vi "Main.vi"() -> ()   [LabVIEW 2018, in "Timer Module.lvlib"]
doc: "This template is based off of the Queued Message Handler design pattern and the Queued Message Handler project template that ships with LabVIEW.\n\nThe main difference is that the queue is private to this module and communication between modules is performed via Broadcast and Request events.\n\nRequest events are wrapped in public API methods and are handled in the Event Handling Loop (EHL) of this VI. Any module can register for Broadcast events sent by this module. The EHL generates messages based on user interface actions.\n\nThe Message Handling Loop (MHL) processes messages generated by the EHL, or by other messages. The messages are string values, so new messages can be added easily to the Message Cases case structure in the MHL. Each message cluster can also provide an optional value for Message Data, which is a variant that can be converted to whatever message-specific data is required.\n_____\nBased on Delacor QMH Project Template 4.1.0.56."
uses:
  Timer Module.lvlib
  <vilib>/Delacor/Delacor QMH/Libraries/Cloneable Module Admin_class/Delacor_lib_QMH_Cloneable Module Admin.lvclass
  C:/Program Files (x86)/National Instruments/LabVIEW 2018/vi.lib/Delacor/Delacor QMH/Libraries/Module Admin_class/Delacor_lib_QMH_Module Admin.lvclass
  Module Data--cluster.ctl
  <vilib>/Delacor/Delacor QMH/Libraries/Cloneable Module Admin_class/Delacor_lib_QMH_Cloneable Module Admin.lvclass/Delacor_lib_QMH_Cloneable Module Admin.ctl
  Stop Argument--cluster.ctl
  <vilib>/Delacor/Delacor QMH/Libraries/Module Admin_class/Delacor_lib_QMH_Module Admin.lvclass/Delacor_lib_QMH_Module Admin.ctl
  Start Timer Argument--cluster.ctl
  <vilib>/Utility/miscctls.llb/LVPointTypeDef.ctl
  <vilib>/Delacor/Delacor QMH/Libraries/Cloneable Module Admin_class/Delacor_lib_QMH_Get Module ID.vi
  <vilib>/Delacor/Delacor QMH/Libraries/Module Admin_class/Delacor_lib_QMH_Get External Launch.vi
  <vilib>/Delacor/Delacor QMH/Libraries/Message Queue_class/Delacor_lib_QMH_Enqueue Message (Single).vi
  <vilib>/Utility/error.llb/Error Cluster From Error Code.vi
  <vilib>/ErrorRing/Error Ring.xnode
  <vilib>/Delacor/Delacor QMH/Libraries/Message Queue_class/Delacor_lib_QMH_Message Queue.lvclass
  Clone Registration/Clone Registration.lvlib
panel:
  out "Timer":timestamp format="%^<%H:%M:%S%3u>T"
  out "error out":errorcluster
  in  "Module Admin":refnum<class "Delacor_lib_QMH_Cloneable Module Admin.lvclass">
  out "Status":string
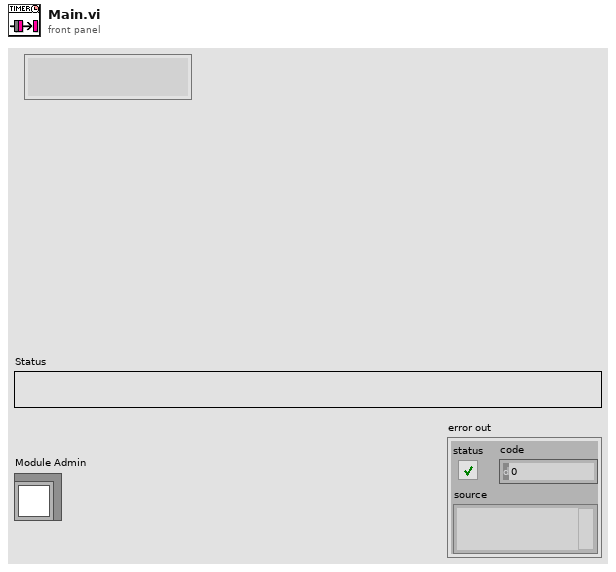
[diagram p1: front panel]
types:
  T1 = typedef "Timer Module.lvlib/Request Events--cluster.ctl" = cluster{"Stop Module":refnum<user-event>, "Show Panel":refnum<user-event>, "Hide Panel":refnum<user-event>, "Show Diagram":refnum<user-event>, "Get Module Execution Status":refnum<user-event>, "Start Timer":refnum<user-event>, "Pause Timer":refnum<user-event>, "Unpause Timer":refnum<user-event>}
  T2 = typedef "Timer Module.lvlib/Module Data--cluster.ctl" = cluster{"Status":string}
  T3 = enum32{"invalid lock state", "Not Locked", "Locked (No Password)", "Password-protected"}
  T4 = typedef "Timer Module.lvlib/Stop Argument--cluster.ctl" = cluster{"Module ID":i32, "Origin":string, "Exit via Stop Module Req?":bool, "Wait for Module to stop?":bool}
  T5 = typedef "Timer Module.lvlib/Start Timer Argument--cluster.ctl" = cluster{"Module ID":i32, "Boolean":bool}
  T6 = typedef "LVPointTypeDef.ctl" = cluster{"Horizontal":i16, "Vertical":i16}
  T7 = enum32{"Invalid", "Standard", "Closed", "Hidden", "Minimized", "Maximized"}
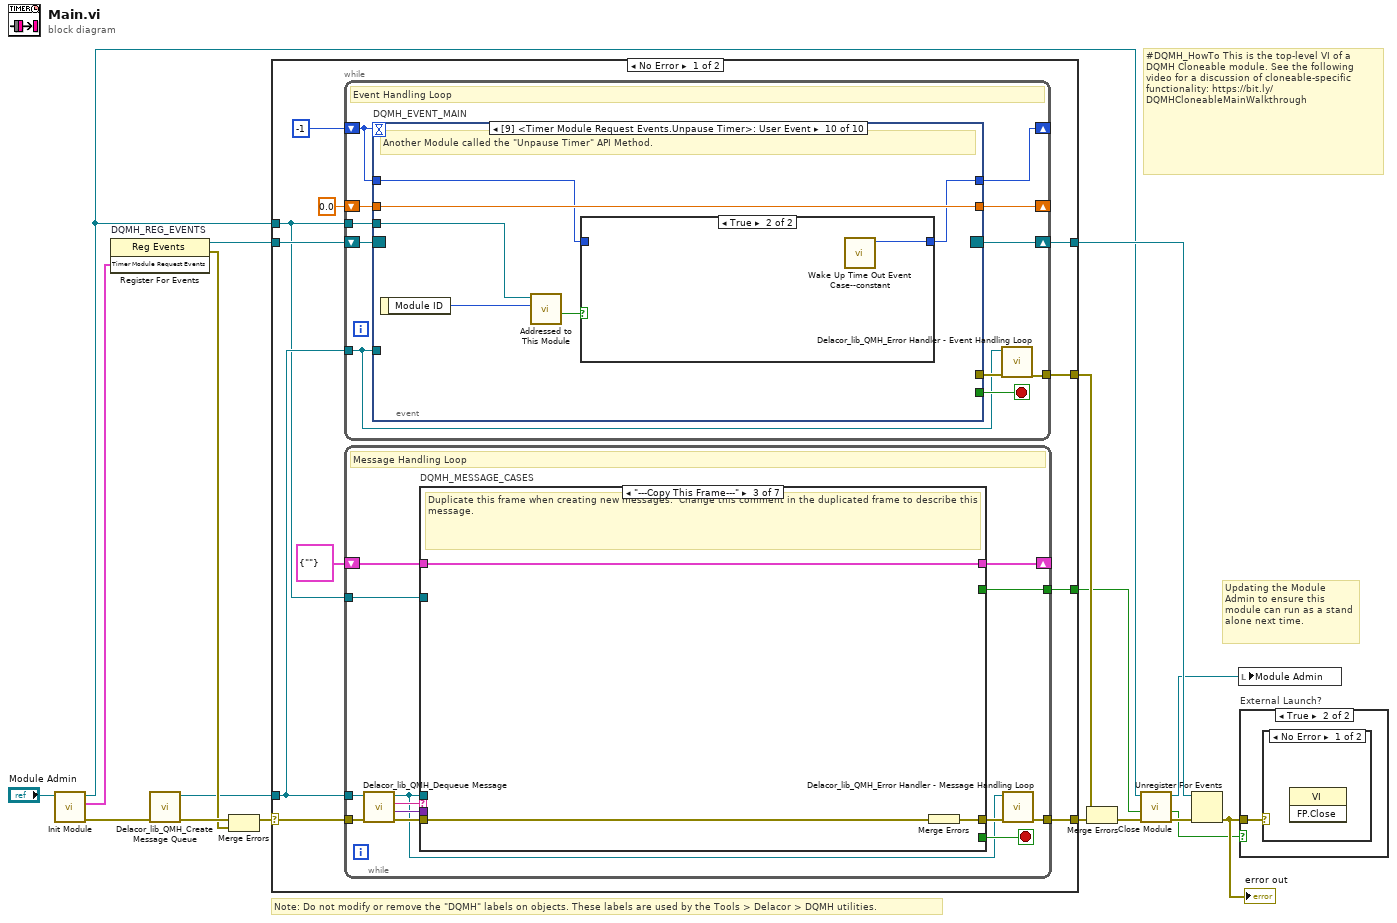
[diagram p0: block diagram]
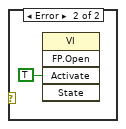
[diagram p3: hidden frame]
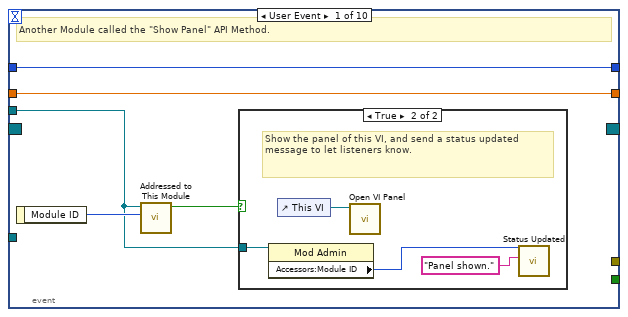
[diagram p4: hidden frame]
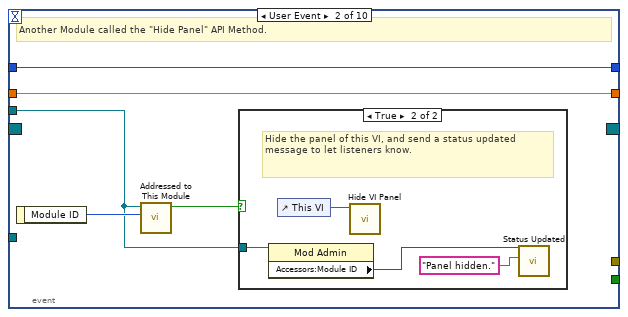
[diagram p6: hidden frame]
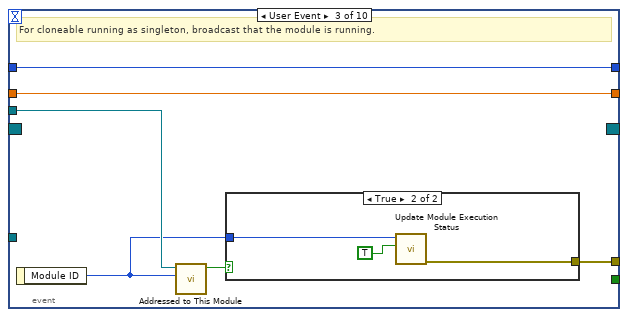
[diagram p8: hidden frame]
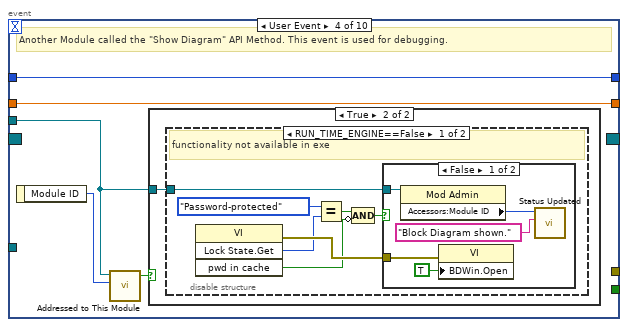
[diagram p10: hidden frame]
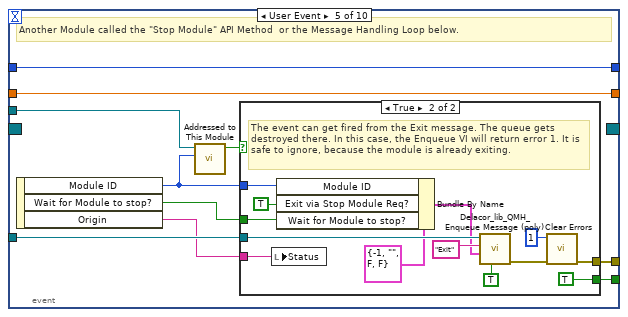
[diagram p14: hidden frame]
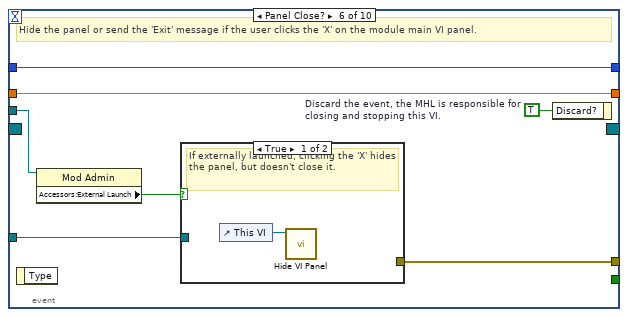
[diagram p16: hidden frame]
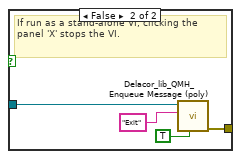
[diagram p17: hidden frame]
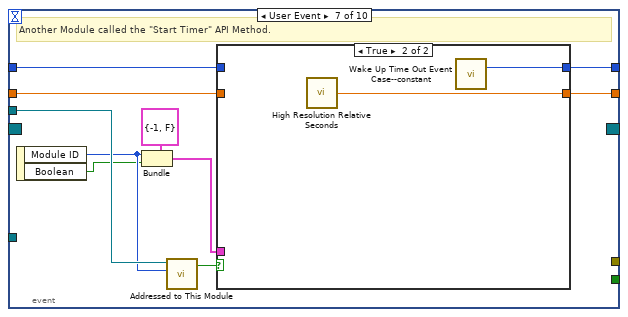
[diagram p18: hidden frame]
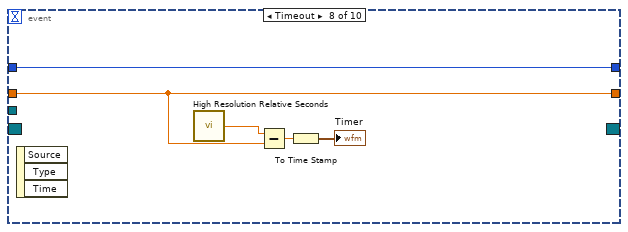
[diagram p20: hidden frame]
diagram:
  # "#DQMH_HowTo This is the top-level VI of a DQMH Cloneable module. See the following video for a discussion of cloneable-specific functionality: https://bit.ly/DQMHCloneableMainWalkthrough"
  # "Note: Do not modify or remove the \"DQMH\" labels on objects. These labels are used by the Tools > Delacor > DQMH utilities."
  # "Updating the Module Admin to ensure this module can run as a stand alone next time."
  n1 = call "Init Module.vi"("Cloneable Module Admin in"="Module Admin") -> ("error out"=w15:errorcluster, "Timer Module Request Events"=w7:T1, "Cloneable Module Admin out"=w4:refnum<class "Delacor_lib_QMH_Cloneable Module Admin.lvclass">)  [unwired: 8 in]
  n2 = register-events "DQMH_REG_EVENTS"(w7) -> (reference out=w8:refnum<event-registration>, error out=w10:errorcluster)  [unwired: 2 in]
  n3 = call <vilib>:"Delacor_lib_QMH_Create Message Queue.vi"("error in (no error)"=w15) -> ("error out"=w12:errorcluster, "Message Queue"=w6:refnum<class "Delacor_lib_QMH_Message Queue.lvclass">)  [unwired: 9 in]
  n4 = Merge Errors(w12, w10) -> (w11:errorcluster)
  n5 = case shown="No Error" w11 {
    selector: w11 -> [w27 w253]
    tunnel: [w29 w253] -> w16
    tunnel: [w26 w252] -> w9
    tunnel: w8 -> [w24 w252]
    tunnel: w6 -> [w23 _]
    tunnel: [w28 _] -> w17
    tunnel: w4 -> [w22 w248]
    tunnel: [w21 _] -> w2
    frame No Error {
      n6 = while {
        tunnel: w23 -> [w34]
        shift-right: [w37] -> w26
        shift-left: w24 -> [w38]
        tunnel: [w39] -> w28
        tunnel: w22 -> [w35]
        shift-right: [w33] -> _
        shift-left: -1 -> [w32]
        shift-right: [w31] -> _
        shift-left: 0.0 ("relative seconds") -> [w30]
        stop <- w36 stop-if-true
        # "Event Handling Loop"
        n7 = event "DQMH_EVENT_MAIN" shown="[9] <Timer Module Request Events.Unpause Timer>: User Event" {
          selector: w38 -> [_ _ _ _ _ _ _ _ _ _]
          dyn-events: [_ _ _ _ _ _ _ _ _ _] -> w37
          timeout: w32 -> [_ _ _ _ _ _ _ _ _ _]
          tunnel: [_ _ _ _ w91 _ _ _ _ _] -> w36
          tunnel: w34 -> [_ _ _ _ w94 w112 _ _ _ _]
          tunnel: [_ _ w64 _ w95 w115 _ _ _ _] -> w40
          tunnel: w35 -> [w43 w52 w62 w70 w93 w113 w129 _ w143 w151]
          tunnel: [w42 w51 w60 w69 w87 w110 w123 w139 w140 w148] -> w33
          tunnel: w32 -> [w42 w51 w60 w69 w87 w110 w124 w139 w141 w149]
          tunnel: [w41 w50 w59 w68 w86 w109 w122 w137 w145 w153] -> w31
          tunnel: w30 -> [w41 w50 w59 w68 w86 w109 w121 w137 w145 w153]
          event User Event {
            # "Another Module called the \"Show Panel\" API Method."
            n8 = event-data() -> ("Module ID"=w44:i32)  [unwired: 1 in]
            n9 = call "Addressed to This Module.vi"("Module ID from Argument"=w44, "Module Admin"=w43) -> ("Addressed to this instance?"=w45:bool)  [unwired: 8 in, 1 out]
            n10 = case shown="True" w45 {
              tunnel: w43 -> [_ w47]
              frame False {
              }
              frame True {
                # "Show the panel of this VI, and send a status updated message to let listeners know."
                n11 = property class="Mod Admin"(reference=w47) -> ("Accessors:Module ID"=w46:i32)  [unwired: 1 in, 2 out]
                n12 = control-ref of="This VI"() -> (w49:refnum<vi>)
                n13 = call "Open VI Panel.vi"("VI"=w49) -> ()  [unwired: 10 in, 1 out]
                n14 = call "Status Updated.vi"("Status"="Panel shown." ("format string"), "Module ID"=w46) -> ()  [unwired: 9 in, 1 out]
              }
            }
          }
          event User Event {
            # "Another Module called the \"Hide Panel\" API Method."
            n15 = event-data() -> ("Module ID"=w53:i32)  [unwired: 1 in]
            n16 = call "Addressed to This Module.vi"("Module ID from Argument"=w53, "Module Admin"=w52) -> ("Addressed to this instance?"=w54:bool)  [unwired: 8 in, 1 out]
            n17 = case shown="True" w54 {
              tunnel: w52 -> [_ w56]
              frame False {
              }
              frame True {
                # "Hide the panel of this VI, and send a status updated message to let listeners know."
                n18 = property class="Mod Admin"(reference=w56) -> ("Accessors:Module ID"=w55:i32)  [unwired: 1 in, 2 out]
                n19 = control-ref of="This VI"() -> (w58:refnum<vi>)
                n20 = call "Hide VI Panel.vi"("VI"=w58) -> ()  [unwired: 10 in, 1 out]
                n21 = call "Status Updated.vi"("Status"="Panel hidden." ("format string"), "Module ID"=w55) -> ()  [unwired: 9 in, 1 out]
              }
            }
          }
          event User Event {
            # "For cloneable running as singleton, broadcast that the module is running."
            n22 = event-data() -> ("Module ID"=w61:i32)  [unwired: 1 in]
            n23 = call "Addressed to This Module.vi"("Module ID from Argument"=w61, "Module Admin"=w62) -> ("Addressed to this instance?"=w63:bool)  [unwired: 8 in, 1 out]
            n24 = case shown="True" w63 {
              tunnel: [_ w67] -> w64
              tunnel: w61 -> [_ w66]
              frame False {
              }
              frame True {
                n25 = call "Update Module Execution Status.vi"("Running?"=TRUE, "Module ID"=w66) -> ("error out"=w67:errorcluster)  [unwired: 9 in]
              }
            }
          }
          event User Event {
            # "Another Module called the \"Show Diagram\" API Method. This event is used for debugging."
            n26 = event-data() -> ("Module ID"=w71:i32)  [unwired: 1 in]
            n27 = call "Addressed to This Module.vi"("Module ID from Argument"=w71, "Module Admin"=w70) -> ("Addressed to this instance?"=w72:bool)  [unwired: 8 in, 1 out]
            n28 = case shown="True" w72 {
              tunnel: w70 -> [_ w73]
              frame False {
              }
              frame True {
                n29 = disable-structure shown="RUN_TIME_ENGINE==False" {
                  disable-tunnel: w73 -> [w74 _]
                  frame condition #0 (active) {
                    # "functionality not available in exe"
                    n30 = invoke class="VI" method="Lock State.Get"() -> (error out=w80:errorcluster, "Get Lock State"=w79:T3, "pwd in cache"=w76:bool)  [unwired: 4 in, 1 out]
                    n31 = Equal?(x=T3."Password-protected", y=w79) -> (x = y?=w77:bool)
                    n32 = Compound Arithmetic op=AND(w77, invert w76) -> (w75:bool)
                    n33 = case shown="False" w75 {
                      tunnel: w80 -> [w85 _]
                      tunnel: w74 -> [w82 _]
                      frame False {
                        n34 = property class="Mod Admin"(reference=w82) -> ("Accessors:Module ID"=w81:i32)  [unwired: 1 in, 2 out]
                        n35 = property class="VI"(error in=w85, "BDWin.Open"=TRUE ("Block Diagram Window:Open")) -> ()  [unwired: 1 in, 2 out]
                        n36 = call "Status Updated.vi"("Status"="Block Diagram shown." ("format string"), "Module ID"=w81) -> ()  [unwired: 9 in, 1 out]
                      }
                      frame True {
                        # "Password-protected VI, and the password is not in the cache. Do not show the diagram."
                      }
                    }
                  }
                  frame condition #1 {
                  }
                }
              }
            }
          }
          event User Event {
            # "Another Module called the \"Stop Module\" API Method  or the Message Handling Loop below."
            n37 = event-data() -> ("Module ID"=w89:i32, "Wait for Module to stop?"=w90:bool, "Origin"=w88:string)  [unwired: 1 in]
            n38 = call "Addressed to This Module.vi"("Module ID from Argument"=w89, "Module Admin"=w93) -> ("Addressed to this instance?"=w92:bool)  [unwired: 8 in, 1 out]
            n39 = case shown="True" w92 {
              tunnel: [_ w107] -> w95
              tunnel: w94 -> [_ w103]
              tunnel: [_ TRUE] -> w91
              tunnel: w90 -> [_ w98]
              tunnel: w89 -> [_ w100]
              tunnel: w88 -> [_ w96]
              frame False {
              }
              frame True {
                # "The event can get fired from the Exit message. The queue gets destroyed there. In this case, the Enqueue VI will return error 1. It is safe to ignore, because the module is already exiting."
                n40 = local write "Status"(w96) -> ()
                n41 = Bundle By Name(cluster=T4 {"Module ID"=-1, "Origin"="", "Exit via Stop Module Req?"=FALSE, "Wait for Module to stop?"=FALSE} ("Stop Argument"), "Module ID"=w100, "Exit via Stop Module Req?"=TRUE, "Wait for Module to stop?"=w98) -> (w97:T4)
                n42 = call-poly <vilib>:"Delacor_lib_QMH_Enqueue Message (poly).vi"("Priority Message? (F)"=TRUE, "Message Data"=w97, "Message"="Exit", "Message Queue in"=w103) -> ("error out"=w108:errorcluster)  [unwired: 6 in, 1 out]
                n43 = call <vilib>:"Clear Errors.vi"("error in (no error)"=w108, "specific error code to clear (0: all)"=1) -> ("error out"=w107:errorcluster)  [unwired: 4 in, 1 out]
              }
            }
          }
          event Panel Close? {
            w114 = TRUE  # Discard the event, the MHL is responsible for closing and stopping this VI.
            # "Hide the panel or send the 'Exit' message if the user clicks the 'X' on the module main VI panel."
            n44 = event-data() -> ()  [unwired: 1 in, 1 out]
            n45 = property class="Mod Admin"(reference=w113) -> ("Accessors:External Launch"=w111:bool)  [unwired: 1 in, 2 out]
            n46 = case shown="True" w111 {
              tunnel: w112 -> [_ w119]
              tunnel: [_ w120] -> w115
              frame True {
                # "If externally launched, clicking the 'X' hides the panel, but doesn't close it."
                n47 = control-ref of="This VI"() -> (w116:refnum<vi>)
                n48 = call "Hide VI Panel.vi"("VI"=w116) -> ()  [unwired: 10 in, 1 out]
              }
              frame False {
                # "If run as a stand-alone VI, clicking the panel 'X' stops the VI."
                n49 = call-poly <vilib>:"Delacor_lib_QMH_Enqueue Message (poly).vi"("Priority Message? (F)"=TRUE, "Message"="Exit", "Message Queue in"=w119) -> ("error out"=w120:errorcluster)  [unwired: 7 in, 1 out]
              }
            }
            n50 = event-data("Discard?"=w114) -> ()  [unwired: 1 in, 1 out]
          }
          event User Event {
            # "Another Module called the \"Start Timer\" API Method."
            n51 = event-data() -> ("Module ID"=w126:i32, "Boolean"=w125:bool)  [unwired: 1 in]
            n52 = Bundle(cluster=T5 {"Module ID"=-1, "Boolean"=FALSE} ("Start Timer Argument"), "Module ID"=w126, "Boolean"=w125) -> (w127:T5)
            n53 = call "Addressed to This Module.vi"("Module ID from Argument"=w126, "Module Admin"=w129) -> ("Addressed to this instance?"=w130:bool)  [unwired: 8 in, 1 out]
            n54 = case shown="True" w130 {
              tunnel: w127 -> [_ _]
              tunnel: w124 -> [w132 _]
              tunnel: [w132 w134] -> w123
              tunnel: [w131 w133] -> w122
              tunnel: w121 -> [w131 _]
              frame False {
              }
              frame True {
                n55 = call <vilib>:"High Resolution Relative Seconds.vi"() -> ("relative seconds"=w133:dbl)
                n56 = call "Wake Up Time Out Event Case--constant.vi"() -> ("Wake up TimeOut Event Case"=w134:i32)  [unwired: 11 in]
              }
            }
          }
          event Timeout {
            n57 = event-data() -> ()  [unwired: 1 in, 3 out]
            n58 = call <vilib>:"High Resolution Relative Seconds.vi"() -> ("relative seconds"=w138:dbl)
            n59 = Subtract(x=w138, y=w137) -> (x-y=w136:dbl)
            n60 = To Time Stamp(1:w136) -> (0:→"Timer":timestamp)
          }
          event User Event {
            # "Another Module called the \"Pause Timer\" API Method."
            n61 = event-data() -> ("Module ID"=w142:i32)  [unwired: 1 in]
            n62 = call "Addressed to This Module.vi"("Module ID from Argument"=w142, "Module Admin"=w143) -> ("Addressed to this instance?"=w144:bool)  [unwired: 8 in, 1 out]
            n63 = case shown="True" w144 {
              tunnel: w141 -> [w146 _]
              tunnel: [w146 w147] -> w140
              frame False {
              }
              frame True {
                w147 = -1  # Put TimeOut event case to sleep
              }
            }
          }
          event User Event {
            # "Another Module called the \"Unpause Timer\" API Method."
            n64 = event-data() -> ("Module ID"=w150:i32)  [unwired: 1 in]
            n65 = call "Addressed to This Module.vi"("Module ID from Argument"=w150, "Module Admin"=w151) -> ("Addressed to this instance?"=w152:bool)  [unwired: 8 in, 1 out]
            n66 = case shown="True" w152 {
              tunnel: [w154 w155] -> w148
              tunnel: w149 -> [w154 _]
              frame False {
              }
              frame True {
                n67 = call "Wake Up Time Out Event Case--constant.vi"() -> ("Wake up TimeOut Event Case"=w155:i32)  [unwired: 11 in]
              }
            }
          }
        }
        n68 = call-dynamic "Delacor_lib_QMH_Error Handler - Event Handling Loop.vi"("error in (no error)"=w40, "Message Queue in"=w34) -> ("dup error in"=w39:errorcluster)  [unwired: 8 in, 1 out]
      }
      n69 = while {
        tunnel: w23 -> [w159]
        shift-right: [w163] -> _
        shift-left: T2 {"Status"=""} ("Data Cluster") -> [w164]
        tunnel: w27 -> [w167]
        tunnel: [w165] -> w29
        tunnel: w22 -> [w157]
        tunnel: [w156] -> w21
        stop <- w162 stop-if-true
        # "Message Handling Loop"
        n70 = call-dynamic "Delacor_lib_QMH_Dequeue Message.vi"("error in (no error)"=w167, "Message Queue in"=w159) -> ("error out"=w166:errorcluster, "Message Data"=w160:variant, "Message"=w161:string, "Message Queue out"=w158:refnum<class "Delacor_lib_QMH_Message Queue.lvclass">)  [unwired: 6 in]
        n71 = case "DQMH_MESSAGE_CASES" shown="\"---Copy This Frame---\"" w161 {
          selector: w161 -> [_ _ _ _ _ _ w233]
          tunnel: w158 -> [_ _ _ _ w197 w223 _]
          tunnel: w166 -> [w187 w191 w194 w196 w207 w229 w235]
          tunnel: [w185 w191 w193 w196 w203 w226 w236] -> w168
          tunnel: w164 -> [w178 w190 w192 w195 w202 w222 w234]
          tunnel: [w177 w190 w192 w195 w202 w222 w234] -> w163
          tunnel: [_ _ _ _ _ w221 _] -> w162
          tunnel: w160 -> [_ _ _ _ w201 w219 _]
          tunnel: w157 -> [w172 _ _ _ w200 w215 w231]
          tunnel: [_ _ _ _ _ w217 _] -> w156
          frame "Initialize" {
            w169 = "Initial Message" ("Initial Message")
            # "#CodeNeeded - Initialize the appearance of the front panel."
            # "#CodeNeeded - Initialize your state data here."
            # "Initialize - Any operation that needs to be done before the module can receive messages. Synchronize Caller Events.vi will inform Start Module.vi that the module has launched and is ready to receive messages. Module Did Init.vi will broadcast that the module initialized."
            n72 = call "Synchronize Caller Events.vi"("error in (no error)"=w187, "Module Admin"=w172) -> ("error out"=w186:errorcluster, "Module Admin out"=w171:refnum<class "Delacor_lib_QMH_Cloneable Module Admin.lvclass">)  [unwired: 8 in]
            n73 = property class="Mod Admin"(reference=w171) -> ("Accessors:Module ID"=w174:i32, "Accessors:External Launch"=w173:bool)  [unwired: 1 in, 2 out]
            n74 = call "Module Name--constant.vi"("Module ID"=w174) -> ("Module Name"=w182:string)  [unwired: 10 in]
            n75 = property class="VI"("Front Panel.Title"=w182) -> (reference out=w184:refnum<vi>, error out=w189:errorcluster)  [unwired: 2 in]
            n76 = Select(t=T7."Hidden" ("State"), s=w173, f=T7."Standard" ("State")) -> (s? t:f=w179:T7)
            n77 = invoke class="VI" method="FP.Open"(reference=w184, error in=w189, "State"=w179) -> (reference out=w183:refnum<vi>, error out=w188:errorcluster)  [unwired: 2 in, 3 out]
            n78 = call "Module Name--constant.vi"("Module ID"=w174) -> ("Module Name"=w175:string)  [unwired: 10 in]
            n79 = Bundle By Name(cluster=w178, "Status"=w169) -> (w177:T2)
            n80 = invoke class="VI" method="FP.Center"(reference=w183, error in=w188) -> ()  [unwired: 1 in, 3 out]
            n81 = property on="Pane" class="Pane"("Origin"=T6 {"Horizontal"=0, "Vertical"=0}) -> ()  [unwired: 2 in, 2 out]
            n82 = call "Module Did Init.vi"("error in (no error)"=w186, "Initialized?"=TRUE, "Origin"=w175, "Module ID"=w174) -> ("error out"=w185:errorcluster)  [unwired: 7 in]
            "Status" <- w169
          }
          frame "--- Module Specific ---" {
            # "Separator -- The following cases handle messages specific to this Module."
          }
          frame "---Copy This Frame---" {
            # "Duplicate this frame when creating new messages.  Change this comment in the duplicated frame to describe this message."
            n83 = Merge Errors(w194) -> (w193:errorcluster)
          }
          frame "--- Exit and Error Handling---" {
            # "Separator - the following cases handle errors and exit messages."
          }
          frame "Error" {
            # "#CodeRecommended - If you ever change the name of this \"Error\" message, you'll need to update the name in the Check Loop Error.vi as well."
            # "#CodeRecommended - If the module is running in standalone mode (External Launch = FALSE), this code will pop up an error dialog and call the 'Exit' message if an error occurs. Add more fine-grained error handling here."
            # "Error - Check the error message data and respond accordingly. This message is sent by the \"Error Handler\" VIs at the end of each loop in this application."
            n84 = property class="Mod Admin"(reference=w200) -> ("Accessors:External Launch"=w198:bool, "Accessors:Module ID"=w199:i32)  [unwired: 1 in, 2 out]
            n85 = Variant To Data(error in=w207, type=errorcluster {"status"=FALSE, "code"=0, "source"=""} ("error constant"), Variant=w201) -> (data=w208:errorcluster, error out=w205:errorcluster)
            n86 = call "Error Reported.vi"("Error"=w208, "Module ID"=w199) -> ()  [unwired: 9 in, 1 out]
            n87 = case shown="False" w198 {
              tunnel: [w213 _] -> w204
              tunnel: w197 -> [w211 _]
              tunnel: w208 -> [w212 _]
              frame False {
                # "If the module is running standalone, then pop up an error dialog and call the \"Exit\" message."
                n88 = call <vilib>:"Simple Error Handler.vi"("error in (no error)"=w212) -> ()  [unwired: 4 in, 5 out]
                n89 = call-poly <vilib>:"Delacor_lib_QMH_Enqueue Message (poly).vi"("Priority Message? (F)"=TRUE, "Message"="Exit", "Message Queue in"=w211) -> ("error out"=w213:errorcluster)  [unwired: 7 in, 1 out]
              }
              frame True {
                # "If the module was launched externally, calling the Error Reported broadcast VI is the only action performed by the \"Error\" message. The module's caller can then process the error appropriately."
              }
            }
            n90 = Merge Errors(w205, w204) -> (w203:errorcluster)
            n91 = local write "error out"(w203) -> ()
          }
          frame "Exit" {
            w220 = 91  # 91: not all Exit messages will have an argument
            w221 = TRUE  # Stop the VI
            # "Release the message queue reference"
            # "#CodeNeeded - Add any required cleanup code here."
            # "Exit - Exit the application."
            n92 = Variant To Data(error in=w229, type=T4 {"Module ID"=-1, "Origin"="", "Exit via Stop Module Req?"=FALSE, "Wait for Module to stop?"=FALSE} ("Stop Argument"), Variant=w219) -> (data=w216:T4, error out=w224:errorcluster)
            n93 = call <vilib>:"Clear Errors.vi"("error in (no error)"=w224, "specific error code to clear (0: all)"=w220) -> ("error out"=w228:errorcluster)  [unwired: 4 in, 1 out]
            n94 = control-ref of="This VI"() -> (w214:refnum<vi>)
            n95 = call-dynamic "Delacor_lib_QMH_Release Message Queue.vi"("error in (no error)"=w228, "Message Queue"=w223) -> ("error out"=w227:errorcluster)  [unwired: 9 in]
            n96 = call "Handle Exit.vi"("Stop Argument"=w216, "Module Admin in"=w215, "VI reference"=w214) -> ("error out"=w225:errorcluster, "Wait for Stop?"=w217:bool)  [unwired: 7 in]
            n97 = Merge Errors(w227, w225) -> (w226:errorcluster)
          }
          frame Default {
            # "'Default' case only runs if there is a message that isn't defined in any of the other cases.  Output a programming error."
            n98 = property class="Mod Admin"(reference=w231) -> ("Accessors:Module ID"=w230:i32)  [unwired: 1 in, 2 out]
            n99 = call "Module Name--constant.vi"("Module ID"=w230) -> ("Module Name"=w232:string)  [unwired: 10 in]
            n100 = xnode "Error Ring"("parameter 0"=w233, "parameter 1"=w232) -> ("error out"=w237:errorcluster)
            n101 = Merge Errors(w235, w237) -> (w236:errorcluster)
          }
        }
        n102 = call-dynamic "Delacor_lib_QMH_Error Handler - Message Handling Loop.vi"("error in (no error)"=w168, "Message Queue in"=w158) -> ("dup error in"=w165:errorcluster)  [unwired: 8 in, 1 out]
      }
    }
    frame Error {
      n103 = call "Synchronize Caller Events.vi"("Module Admin"=w248) -> ("Module Admin out"=w247:refnum<class "Delacor_lib_QMH_Cloneable Module Admin.lvclass">)  [unwired: 9 in, 1 out]
      n104 = property class="Mod Admin"(reference=w247) -> ("Accessors:Module ID"=w246:i32)  [unwired: 1 in, 2 out]
      n105 = call "Module Name--constant.vi"("Module ID"=w246) -> ("Module Name"=w251:string)  [unwired: 10 in]
      n106 = call "Remove.vi"("Module ID"=w246) -> ()  [unwired: 9 in, 2 out]
      n107 = Format Into String(format string="An error occurred during initialization. %s is no longer running.", w251) -> (resulting string=w249:string)  [unwired: 2 in, 1 out]
      n108 = call "Error Reported.vi"("Additional Information"=w249, "Error"=w253, "Module ID"=w246) -> ()  [unwired: 8 in, 1 out]
    }
  }
  n109 = Merge Errors(w17, w16) -> (w18:errorcluster)
  n110 = call "Close Module.vi"("error in (no error)"=w18, "Wait for stop?"=w2, "Module Admin in"=w4) -> ("error out"=w14:errorcluster, "External Launch"=w1:bool, "Module Admin out"=w3:refnum<class "Delacor_lib_QMH_Cloneable Module Admin.lvclass">)  [unwired: 6 in]
  n111 = Unregister For Events(event registration refnum=w9, error in=w14) -> (error out=w13:errorcluster)
  "error out" <- w13
  n112 = local write "Module Admin"(w3) -> ()
  n113 = case "External Launch?" shown="True" w1 {
    tunnel: w13 -> [_ w254]
    frame False {
    }
    frame True {
      n114 = case shown="No Error" w254 {
        frame No Error {
          n115 = invoke class="VI" method="FP.Close"() -> ()  [unwired: 3 in, 3 out]
        }
        frame Error {
          n116 = invoke class="VI" method="FP.Open"("Activate"=TRUE ("Activate?")) -> ()  [unwired: 4 in, 5 out]
        }
      }
    }
  }
